vi "UMB_Tend Straight.vi"(11 "behavior weights":i8[](array[numeric])=[0, 1, 0]) -> (3 "Behavior Output":T1={"Goodness"=[0, 0, 0, 0, 0, 0, 0, 1, 0, 0, 0, 0, 0, 0, 0], "Velocity"=[7, 7, 7, 7, 7, 7, 7, 8, 7, 7, 7, 7, 7, 7, 7], "Weight"=1})   [LabVIEW 2012]
uses:
  NINJA Code/Tugboat/Robo_Programs/behaviorOutput_t.ctl
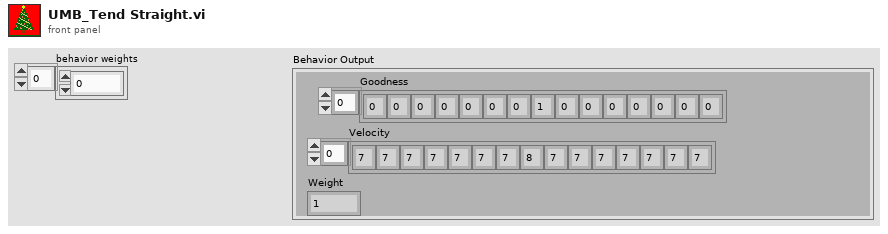
[diagram p1: front panel]
types:
  T1 = typedef "behaviorOutput_t.ctl" = cluster{"Goodness":i8[], "Velocity":i8[], "Weight":i8}
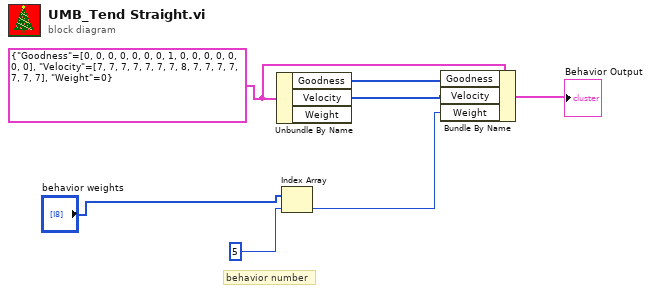
[diagram p0: block diagram]
diagram:
  w6 = T1 {"Goodness"=[0, 0, 0, 0, 0, 0, 0, 1, 0, 0, 0, 0, 0, 0, 0], "Velocity"=[7, 7, 7, 7, 7, 7, 7, 8, 7, 7, 7, 7, 7, 7, 7], "Weight"=0} ("Behavior Output")
  # "behavior number"
  n1 = Unbundle By Name(w6) -> ("Goodness"=w7:i8[], "Velocity"=w4:i8[])  [unwired: 1 out]
  n2 = Index Array(array="behavior weights", index=5) -> (element=w1:i8)
  n3 = Bundle By Name(cluster=w6, "Goodness"=w7, "Velocity"=w4, "Weight"=w1) -> (→"Behavior Output":T1)
